vi "DataGrabber.vi"(0 "# Images In":u16=208 min=1 max=10000, 1 "Camera Handle":u32=16842752, 2 "error in (no error)":errorcluster) -> (3 "# Images Out":u16, 4 "Camera Handle":u32, 5 "Data":dbl[][](array[numeric]), 6 "error out":errorcluster)   [LabVIEW 2013]
panel:
  out "Data Graph":sgl[][](graph)
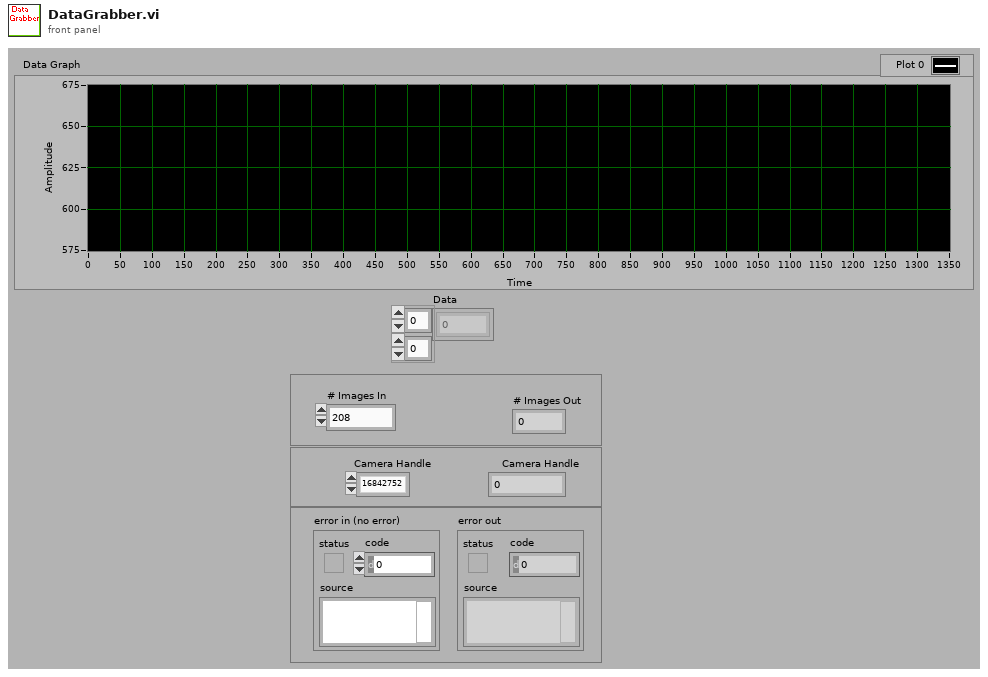
[diagram p1: front panel]
types:
  T1 = cluster{"Camera Handle":u32, "Pulser Handle":u32, "File Handle":u32, "Display Handle":u32, "Image Handle":u32}
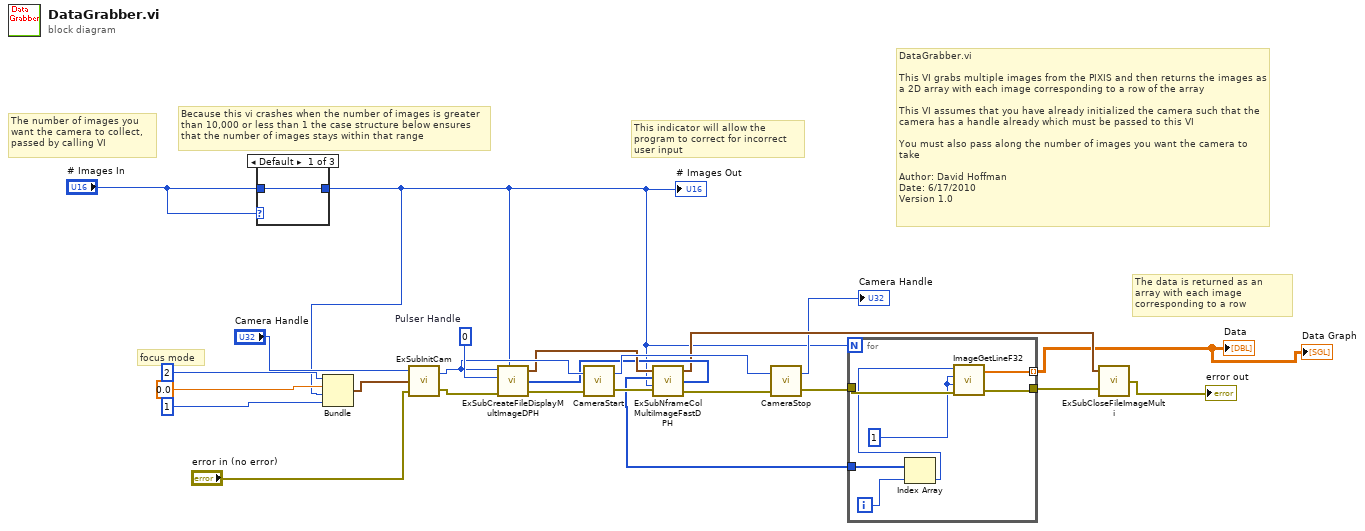
[diagram p0: block diagram]
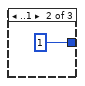
[diagram p2: hidden frame]
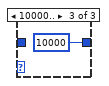
[diagram p3: hidden frame]
diagram:
  w19 = u32 0  # Pulser Handle
  # "This indicator will allow the program to correct for incorrect user input"
  # "Because this vi crashes when the number of images is greater than 10,000 or less than 1 the case structure below ensures that the number of images stays within that range"
  # "The data is returned as an array with each image corresponding to a row"
  # "DataGrabber.vi\n\nThis VI grabs multiple images from the PIXIS and then returns the images as a 2D array with each image corresponding to a row of the array\n\nThis VI assumes that you have already initialized the camera such that the camera has a handle already which must be passed to this VI\n\nYou must also pass along the number of images you want the camera to take\n\nAuthor: David Hoffman\nDate: 6/17/2010\nVersion 1.0"
  # "The number of images you want the camera to collect, passed by calling VI"
  # "focus mode"
  n1 = case shown="Default" "# Images In" {
    tunnel: [w25 u16 1 u16 10000] -> w2
    tunnel: "# Images In" -> [w25 _ _]
    frame Default {
    }
    frame ..1 {
    }
    frame 10000.. {
    }
  }
  "# Images Out" <- w2
  n2 = Bundle(u32 2, 0.0, "# Images In"=w2, u32 1) -> (w21:cluster{u32, dbl, "# Images In":u16, u32})  [unwired: 1 in]
  n3 = call "ExSubInitCam.vi"("error in (no error)"="error in (no error)", "Camera Information"=w21, "Camera Handle"="Camera Handle") -> ("error out"=w20:errorcluster, "Camera Handle"=w18:u32)
  n4 = call "ExSubCreateFileDisplayMultImageDPH.vi"("Camera Handle"=w18, "Pulser Handle"=w19, "error in (no error)"=w20, "Number of Images"=w2) -> ("Handles Out"=w13:T1, "Array"=w12:u32[], "error out"=w17:errorcluster)  [unwired: 1 in]
  n5 = call <userlib>:"CameraStart.vi"("error in"=w17, "Camera Handle"=w18) -> ("error out"=w16:errorcluster, "Camera Handle"=w14:u32)
  n6 = call "ExSubNframeColMultiImageFastDPH.vi"("image handles"=w12, "error in (no error)"=w16, "Number of Images"=w2, "Handle Cluster"=w13) -> ("error out"=w15:errorcluster, "Handle Cluster"=w9:T1, "data handles"=w8:u32[])
  n7 = call <userlib>:"CameraStop.vi"("error in"=w15, "Camera Handle"=w14) -> ("error out"=w11:errorcluster, "Camera Handle"=→"Camera Handle":u32)
  n8 = for {
    N: w2 -> [_]
    tunnel: w11 -> [w34]
    tunnel: w8 -> [w31]
    tunnel: [w29] -> w10
    tunnel: [w28] -> w1 mode=indexing
    i -> [w33]
    w32 = u32 1
    n9 = Index Array(array=w31, index=w33) -> (element=w30:u32)
    n10 = call <userlib>:"ImageGetLineF32.vi"("error in"=w34, "Z Position"=w32, "Y Position"=w32, "Data Handle"=w30) -> ("error out"=w29:errorcluster, "Array F32"=w28:sgl[])  [unwired: 1 out]
  }
  "Data" <- w1
  "Data Graph" <- w1
  n11 = call "ExSubCloseFileImageMulti.vi"("error in (no error)"=w10, "Handles In"=w9) -> ("error out"=→"error out":errorcluster)
